vi "T1 with B Sweep.vi"() -> ()   [LabVIEW 2012]
uses:
  <vilib>/Analysis/1siggen.llb/Ramp Pattern by Samples.vi
  <vilib>/Analysis/NI_AALBase.lvlib
panel:
  in  "Y Parameters":T1={"Number of Y Steps"=200, "Max Y (V)"=2.0, "Min Y (V)"=-2.0}
  in  "X Parameters":T2={"Number of X Steps"=200, "Max X (V)"=2.0, "Min X (V)"=-2.0}
  in  "B samples":i32=128
  in  "B end":dbl=1.0 format="%0.2f"
  in  "B Start":dbl format="%0.2f"
  in  "RS232 settings":cluster{"Portnumber":i32, "Baudrate":u16}={"Portnumber"=12, "Baudrate"=5} {"Portnumber" items=["COM1", "COM2", "COM3", "COM4", "COM5", "COM6", "COM7", "COM8", "COM9", "COM10", "COM11", "COM12", "COM13", "COM14", "COM15", "COM16", "COM17", "COM18", "COM19", "COM20", "COM21", "COM22", "COM23", "COM24", "COM25", "COM26", "COM27", "COM28", "COM29", "COM30"]; "Baudrate" items=["9600", "14400", "19200", "38400", "57600", "115200"]}
  in  "Z Pos":dbl=77.35
  in  "Y pos":dbl=9.0
  in  "X Pos":dbl=41.0
  in  "Tracking Interval":dbl=1.0
  in  "Total Time":dbl=5.0
  in  "Pule Sequence file path":path=path "C:/Users/Ouyang Group/Documents/Data/8-6-15/T1 pulse sequence"
  in  "EPR file path":path=path "C:/Users/Ouyang Group/Documents/Data/8-10-15/test"
  in  "Tab Control":T3(tab)=enum."T1"
  in  "Rate (Hz)":dbl=2.0
  in  "Pulse MW":bool
  in  "Pulse Laser":bool
  in  "Delay Blocks":u16=4
  in  "Divide By":u16(ring) items=["1", "8", "16", "32"]
  in  "MW width Min":dbl=2e-08
  in  "MW width step size":dbl=5e-09
  in  "MW width Max":dbl=5e-07
  in  "Rest time Min":dbl=2e-08
  in  "Rest time Max":dbl=0.0002
  in  "Rest time No. Steps":i32=20
  in  "type":u16(ring)=1 items=["Linear", "Logarithmic"]
  in  "Tau step size":dbl
  in  "Tau max":dbl
  in  "Tau min":dbl
  in  "Rabi Frequency":dbl
  in  "Pulse offset 2":dbl
  in  "Rabi Frequency  2":dbl
  in  "Tau max 2":dbl
  in  "Tau min 2":dbl
  in  "Tau step size 2":dbl
  in  "Equal Pulse length":bool
  in  "Pulse offset":dbl
  in  "Tau":dbl
  in  "Rabi Frequency  3":dbl
  in  "Tau' max 2":dbl
  in  "Tau' min 2":dbl
  in  "Tau' step size 2":dbl
  in  "Rabi Frequency 2":dbl
  in  "Tau min 3":dbl
  in  "Tau max  3":dbl
  in  "Tau step size 3":dbl
  in  "No. Pi Pulses":i32
  in  "Pulse offset 3":dbl
  in  "0->+?":bool
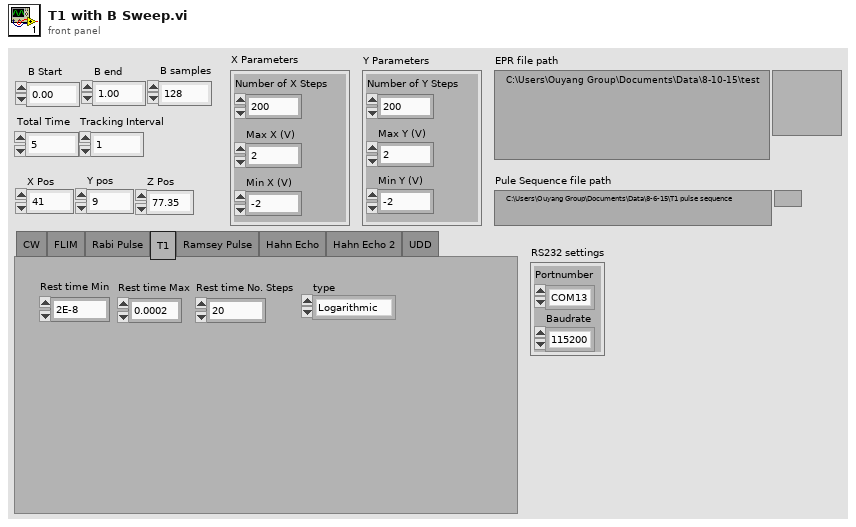
[diagram p1: front panel]
types:
  T1 = cluster{"Number of Y Steps":i32, "Max Y (V)":dbl, "Min Y (V)":dbl}
  T2 = cluster{"Number of X Steps":i32, "Max X (V)":dbl, "Min X (V)":dbl}
  T3 = enum32{"CW", "FLIM", "Rabi Pulse", "T1", "Ramsey Pulse", "Hahn Echo", "Hahn Echo 2", "UDD"}
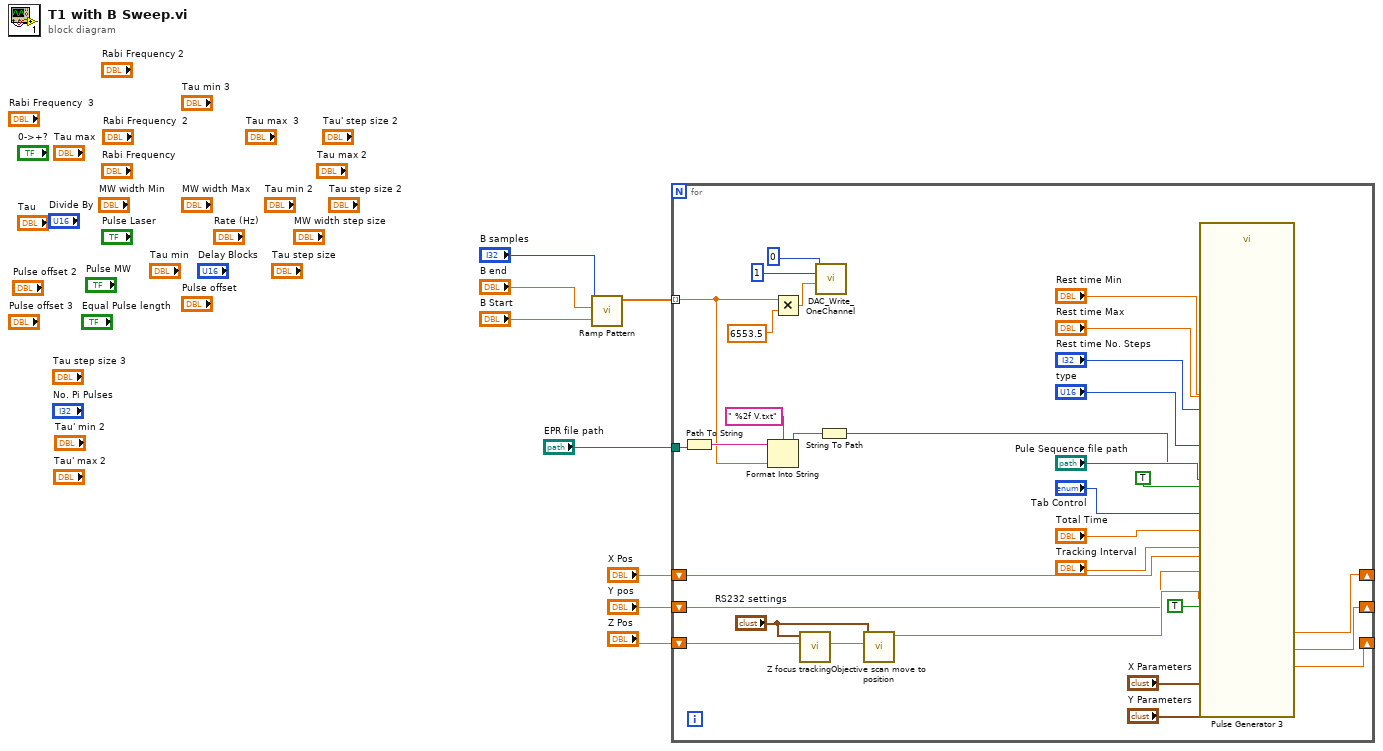
[diagram p0: block diagram]
diagram:
  n1 = call-poly <vilib>:"Ramp Pattern.vi"("start"="B Start", "end"="B end", "samples"="B samples") -> ("Ramp Pattern"=w2:dbl[])  [unwired: 7 in, 1 out]
  n2 = for {
    shift-right: [w24] -> _
    shift-left: "Z Pos" -> [w27]
    shift-right: [w22] -> _
    shift-left: "X Pos" -> [w26]
    shift-right: [w23] -> _
    shift-left: "Y pos" -> [w25]
    tunnel: w2 -> [w9] mode=indexing
    tunnel: "EPR file path" -> [w14]
    n3 = Path To String(path=w14) -> (string=w13:string)
    n4 = Format Into String(format string=" %2f V.txt", initial string=w13, w9) -> (resulting string=w15:string)  [unwired: 1 in, 1 out]
    n5 = Multiply(x=w9, y=6553.5) -> (x*y=w20:dbl)
    n6 = call "Z focus tracking.vi"("Position"=w27, "RS232 settings"="RS232 settings") -> ("center"=w31:dbl)  [unwired: 6 in, 2 out]
    n7 = call "DAC_Write_OneChannel.vi"("Value"=w20, "Channel"=u16 1, "DeviceIndex"=u64 0) -> ()  [unwired: 7 in, 2 out]
    n8 = String To Path(string=w15) -> (path=w12:path)
    n9 = call "Objective scan move to position.vi"("Z position"=w31, "RS232 settings"="RS232 settings") -> ("Z Position 2"=w29:dbl)  [unwired: 9 in]
    n10 = call "Pulse Generator 3.vi"("Total Time"="Total Time", "EPR file path"=w12, "Z Pos"=w29, "Pule Sequence file path"="Pule Sequence file path", "X Pos"=w26, "Y pos"=w25, "track and epr"=TRUE, "Z-track?"=TRUE, "Y Parameters"="Y Parameters", "Tracking Interval"="Tracking Interval", "Tab Control"="Tab Control", "X Parameters"="X Parameters", "Rest time Min"="Rest time Min", "Rest time Max"="Rest time Max", "Rest time No. Steps"="Rest time No. Steps", "type"="type") -> ("Y Position"=w23:dbl, "Z Position"=w24:dbl, "X Position"=w22:dbl)  [unwired: 9 in]
  }
